vi "json.vi"() -> ()   [LabVIEW 2018]
uses:
  694c4d04-db2a-4f9b-98f9-4049c5ef1fde.vi
  <vilib>/JDP Science/JSONtext/JSONtext.lvlib
  <vilib>/JDP Science/JSONtext/Config Files/Config File.lvclass
panel:
  out "changes":refnum<class "Config File.lvclass">
  out "Template Used (file missing or corrupted)":bool
  out "<JSON>Config":string
  out "Config File":refnum<class "Config File.lvclass">
  in  "config file path":path
  out "Rest of Input String":string
  in  "Product Info":T1
  in  "Barcode":string="ADB-12345"
  out "Str JSON":string
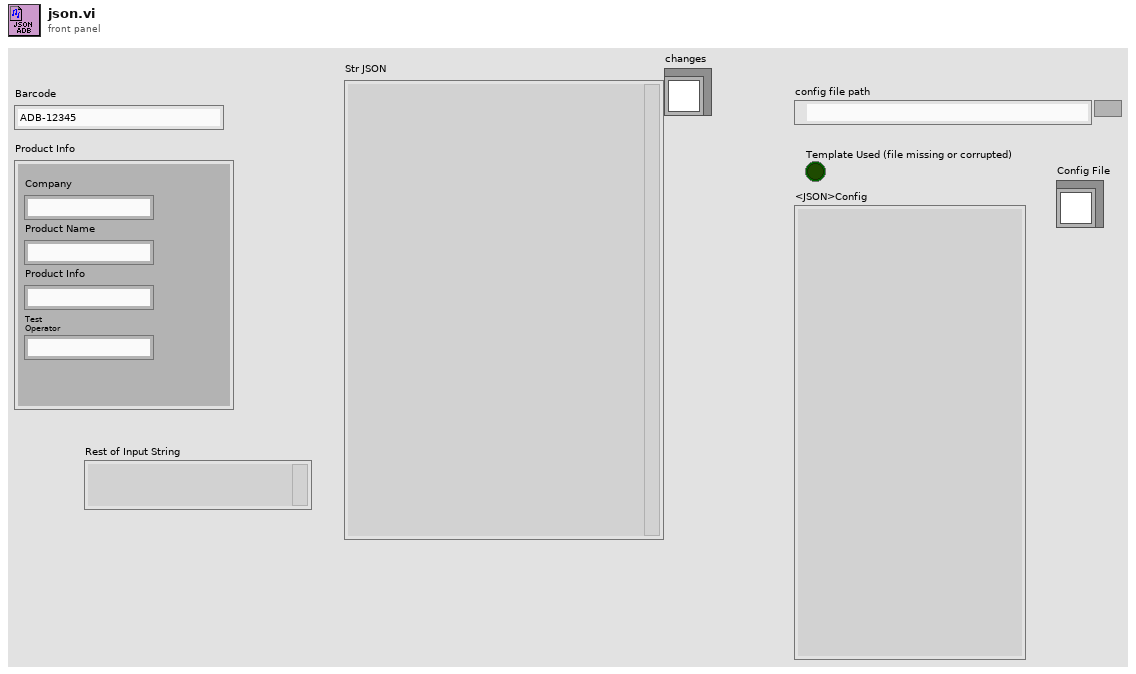
[diagram p1: front panel]
types:
  T1 = cluster{"Company":string, "Product Name":string, "Product Info":string, "Test Operator":string}
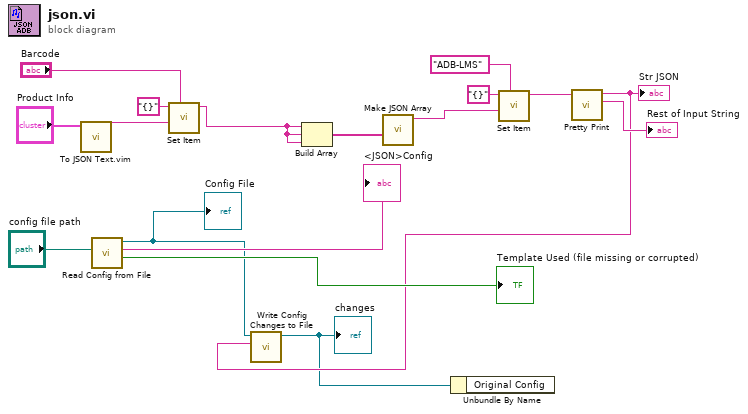
[diagram p0: block diagram]
diagram:
  n1 = call "To JSON Text.vim"("Anything"="Product Info") -> ("<JSON>"=w9:string)  [unwired: 9 in, 1 out]
  n2 = call <vilib>:"Read Config from File.vi"("config file path"="config file path") -> ("Template Used (file missing or corrupted)"=→"Template Used (file missing or corrupted)":bool, "<JSON>Config"=→"<JSON>Config":string, "Config File"=w3:refnum<class "Config File.lvclass">)  [unwired: 7 in, 1 out]
  "Config File" <- w3
  n3 = call <vilib>:"Set Item.vi"("$Path or Item Name"="Barcode", "JSON to Insert"=w9, "JSON"="{}") -> ("<JSON>"=w7:string)  [unwired: 5 in, 2 out]
  n4 = Build Array(w7, w7, w7) -> (w11:string[])
  n5 = call <vilib>:"Make JSON Array.vi"("JSON Elements"=w11) -> ("<JSON>"=w12:string)  [unwired: 9 in, 1 out]
  n6 = call <vilib>:"Set Item.vi"("$Path or Item Name"="ADB-LMS", "JSON to Insert"=w12, "JSON"="{}") -> ("<JSON>"=w15:string)  [unwired: 5 in, 2 out]
  n7 = call <vilib>:"Pretty Print.vi"("JSON"=w15) -> ("Rest of Input String"=→"Rest of Input String":string, "<JSON>"=w2:string)  [unwired: 8 in, 1 out]
  "Str JSON" <- w2
  n8 = call <vilib>:"Write Config Changes to File.vi"("New Config"=w2, "Config File in"=w3) -> ("Config File"=w1:refnum<class "Config File.lvclass">)  [unwired: 6 in, 3 out]
  "changes" <- w1
  n9 = Unbundle By Name(w1) -> ()  [unwired: 1 out]
